vi "Hamming Distance.vi"(1 "LED 2":u8[](array[numeric]) format="0x%02x", 2 "LED 1":u8[](array[numeric]) format="0x%02x") -> (0 "Hamming Distance":u32)   [LabVIEW 2013]
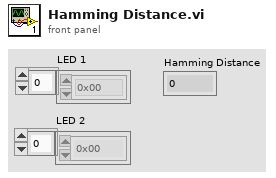
[diagram p1: front panel]
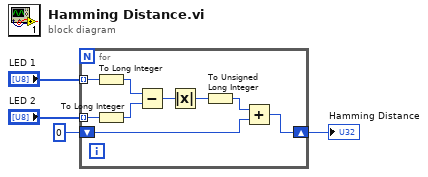
[diagram p0: block diagram]
diagram:
  n1 = for {
    shift-right: [w5] -> w1
    shift-left: u32 0 -> [w6]
    tunnel: "LED 1" -> [w13] mode=indexing
    tunnel: "LED 2" -> [w12] mode=indexing
    n2 = To Long Integer(number=w13) -> (32bit integer=w11:i32)
    n3 = To Long Integer(number=w12) -> (32bit integer=w10:i32)
    n4 = Subtract(x=w11, y=w10) -> (x-y=w9:i32)
    n5 = Absolute Value(x=w9) -> (abs(x)=w8:i32)
    n6 = To Unsigned Long Integer(number=w8) -> (unsigned 32bit integer=w7:u32)
    n7 = Add(x=w7, y=w6) -> (x+y=w5:u32)
  }
  "Hamming Distance" <- w1
